vi "RichToFlatni_measurementlink_measurement_v2_MeasurementDetails.vi"(5 "OutputClusterType":T1, 11 "InputCluster":T2) -> (3 "OutputCluster":T1)   [LabVIEW 2020, in "Measurement Plugin Measurement Service Base V2.lvlib"]
uses:
  Measurement Plugin Measurement Service Base V2.lvlib
  ni_measurementlink_measurement_v2_MeasurementDetails.ctl
  ni_measurementlink_measurement_v2_MeasurementDetails_Flat.ctl
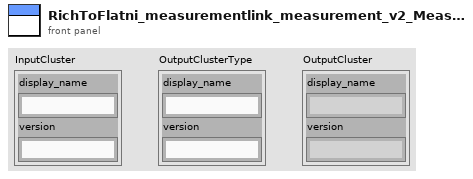
[diagram p1: front panel]
types:
  T1 = typedef "Measurement Plugin Measurement Service Base V2.lvlib/ni_measurementlink_measurement_v2_MeasurementDetails_Flat.ctl" = cluster{"display_name":string, "version":string}
  T2 = typedef "Measurement Plugin Measurement Service Base V2.lvlib/ni_measurementlink_measurement_v2_MeasurementDetails.ctl" = cluster{"display_name":string, "version":string}
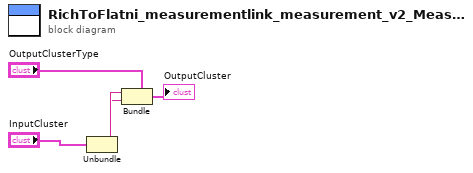
[diagram p0: block diagram]
diagram:
  n1 = Unbundle "Unbundle"("InputCluster") -> ("display_name"=w2:string, "version"=w1:string)
  n2 = Bundle "Bundle"(cluster="OutputClusterType", "display_name"=w2, "version"=w1) -> (→"OutputCluster":T1)
